vi "Plot get control references by name.vi"(8 "error in (no error)":errorcluster, 10 "Control label names":string[](array[string]), 11 "Cluster reference":refnum<vi>) -> (0 "error out":errorcluster, 2 "Controls[]":refnum<vi>[](array[refnum]))   [LabVIEW 2021, in "RocketPlot.lvlib"]
uses:
  RocketPlot.lvlib
  <vilib>/Utility/error.llb/Error Cluster From Error Code.vi
  <vilib>/ErrorRing/Error Ring.xnode
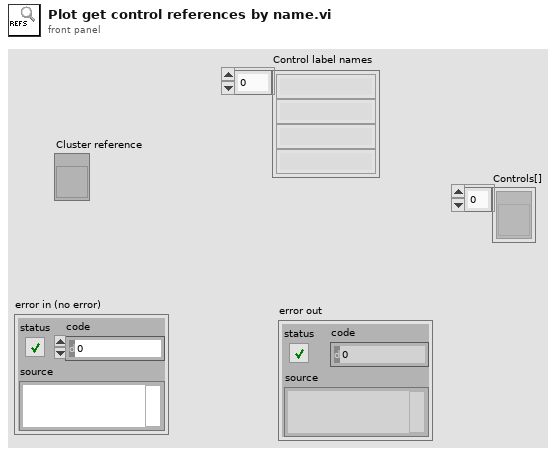
[diagram p1: front panel]
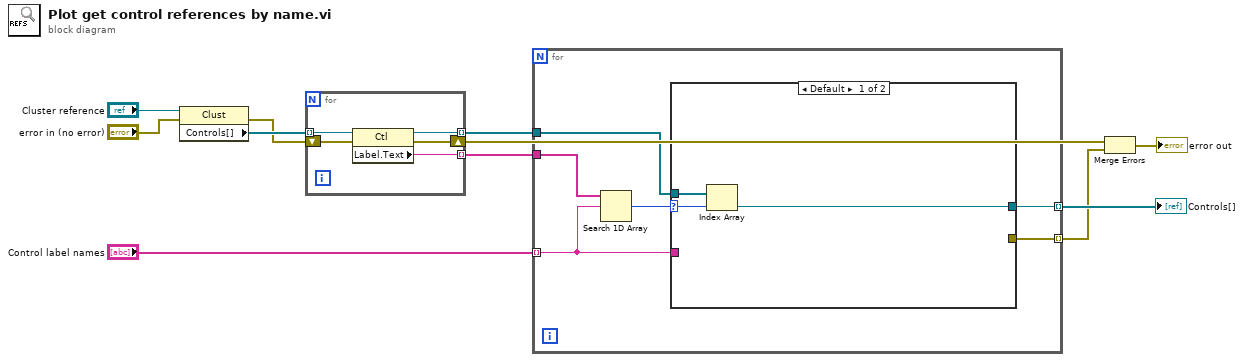
[diagram p0: block diagram]
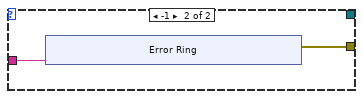
[diagram p2: hidden frame]
diagram:
  n1 = property class="Clust"(reference="Cluster reference", error in="error in (no error)") -> (error out=w6:errorcluster, "Controls[]"=w8:refnum<vi>[])  [unwired: 1 out]
  n2 = for {
    tunnel: w8 -> [w16] mode=indexing
    tunnel: [w15] -> w10 mode=indexing
    tunnel: [w14] -> w11 mode=indexing
    shift-right: [w12] -> w3
    shift-left: w6 -> [w13]
    n3 = property class="Ctl"(reference=w16, error in=w13) -> (reference out=w15:refnum<vi>, error out=w12:errorcluster, "Label.Text"=w14:string)
  }
  n4 = for {
    tunnel: w11 -> [w22]
    tunnel: w10 -> [w20]
    tunnel: "Control label names" -> [w19] mode=indexing
    tunnel: [w18] -> w4 mode=indexing
    tunnel: [w17] -> w2 mode=indexing
    n5 = Search 1D Array(1D array=w22, element=w19) -> (index of element=w21:i32)  [unwired: 1 in]
    n6 = case shown="Default" w21 {
      selector: w21 -> [w25 _]
      tunnel: w19 -> [_ w27]
      tunnel: [_ w26] -> w17
      tunnel: w20 -> [w24 _]
      tunnel: [w23 _] -> w18
      frame Default {
        n7 = Index Array(array=w24, index=w25) -> (element=w23:refnum<vi>)
      }
      frame -1 {
        n8 = xnode "Error Ring"("parameter 0"=w27) -> ("error out"=w26:errorcluster)
      }
    }
  }
  "Controls[]" <- w4
  n9 = Merge Errors(w3, w2) -> (→"error out":errorcluster)
